vi "公式复合写入.vi"(8 "公式":cluster{"X^2":dbl, "X":dbl, "b":dbl}, 9 "量程下拉列表":enum16{"低量程", "高量程"}(ring), 10 "测量模式":T1(ring), 11 "参数下拉列表":u16(ring) items=["总氮"=2]) -> ()   [LabVIEW 2016, in "斯坦道总磷总氮.lvlib"]
uses:
  <vilib>/Utility/miscctls.llb/LVPointTypeDef.ctl
panel:
  in  "读取":bool
  in  "一键写入":bool=TRUE
  out "连接的字符串":string
  in  "关闭":bool
  in  "写入":bool
  # "请选择要写入的参数"
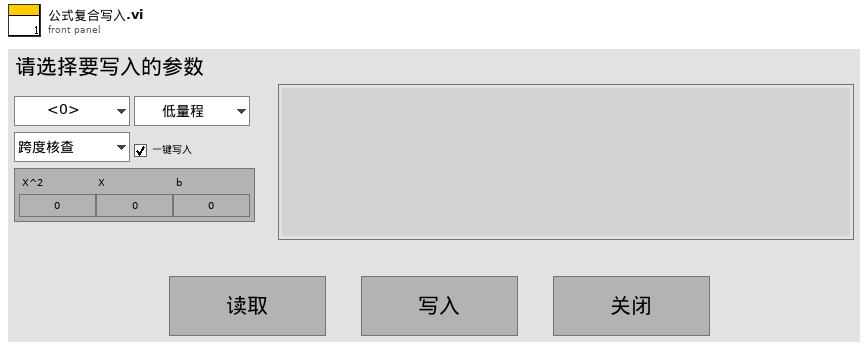
[diagram p1: front panel]
types:
  T1 = enum16{"跨度核查", "水样测量", "零点核查", "标样核查", "加标回收", "快捷测试", "空白校准", "标样校准"}
  T2 = typedef "LVPointTypeDef.ctl" = cluster{"Horizontal":i16, "Vertical":i16}
  T3 = cluster{"系统时间":timestamp, "工作状态":u16, "测量模式":enum16{"待机", "连续模式", "周期模式", "定点模式", "受控模式", "手动模式"}, "告警代码":u16, "故障代码":u16, "日志代码":u16, "软件版本":u16, "F0":sgl, "F1":sgl, "F2":sgl, "F3":sgl, "T":sgl, "H":sgl, "id":u16, "flowid":u16, "量程":u16, "总磷控温温度1":sgl, "营养盐控温温度2":sgl, "ADC":sgl}
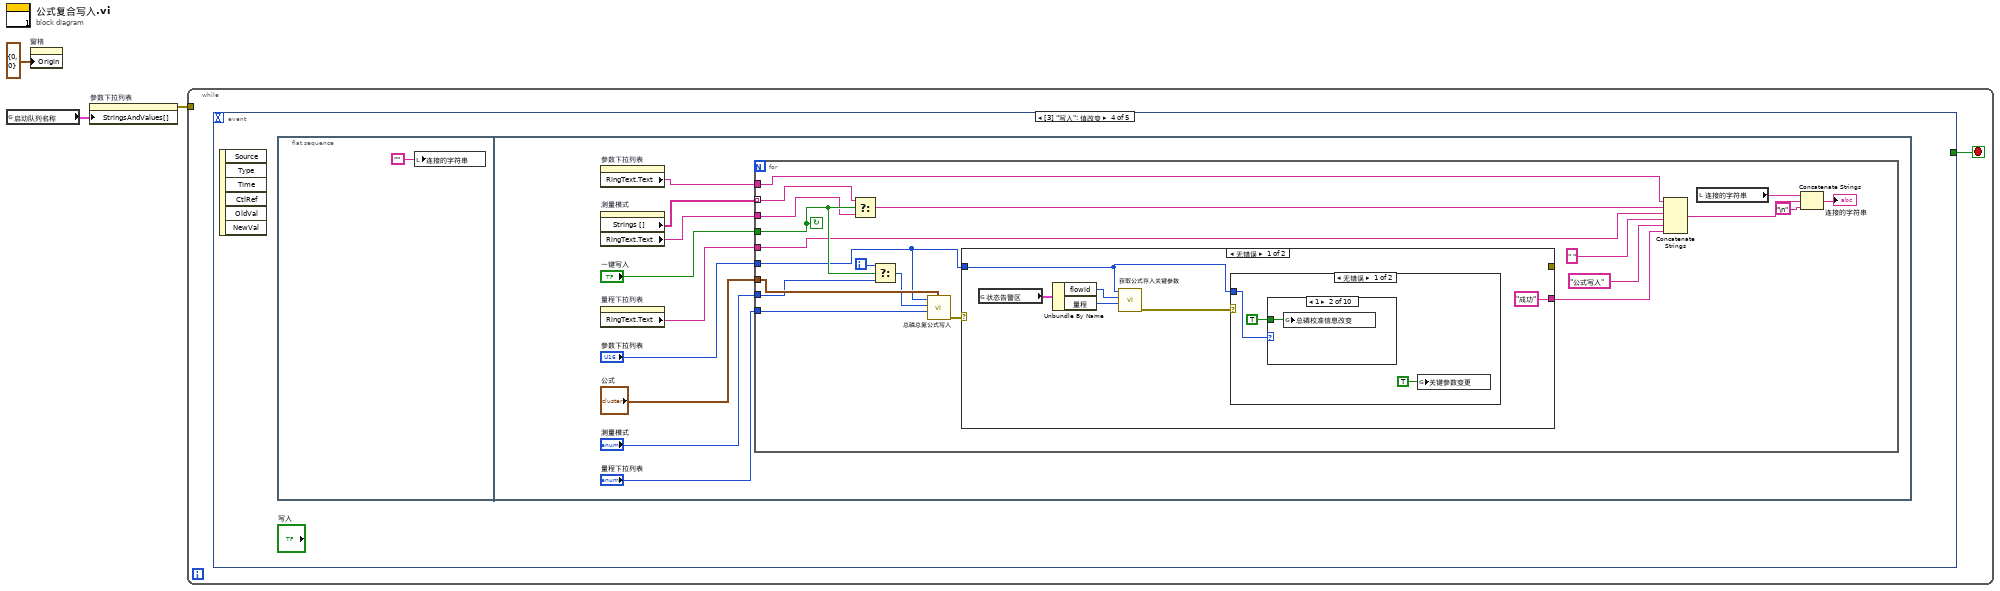
[diagram p0: block diagram]
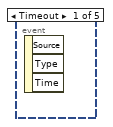
[diagram p2: hidden frame]
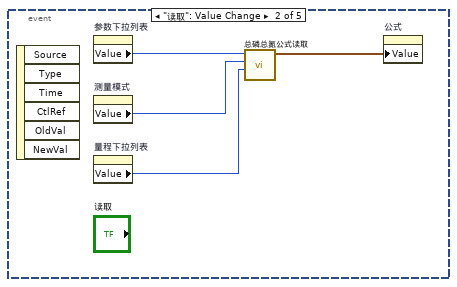
[diagram p3: hidden frame]
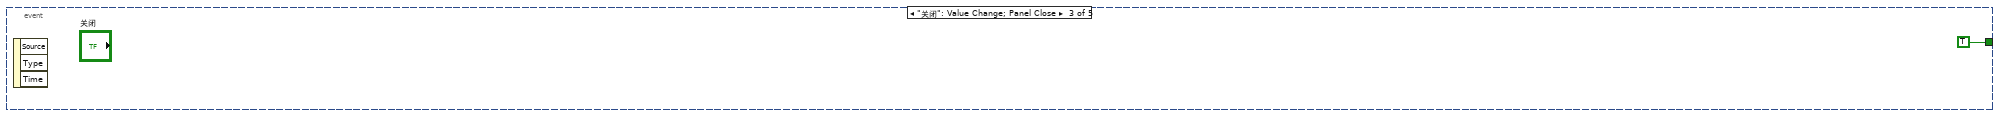
[diagram p4: hidden frame]
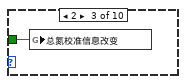
[diagram p6: hidden frame]
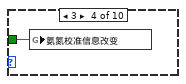
[diagram p7: hidden frame]
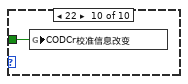
[diagram p13: hidden frame]
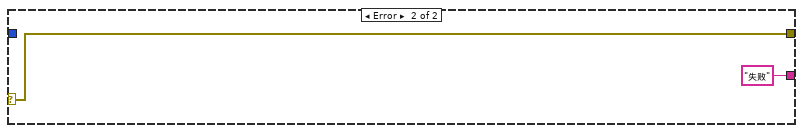
[diagram p15: hidden frame]
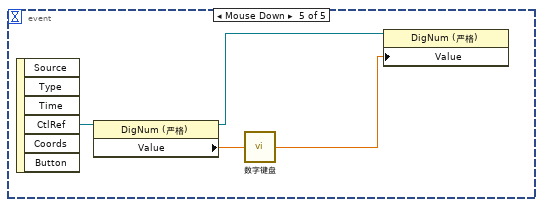
[diagram p16: hidden frame]
diagram:
  n1 = global read "model config var.vi" "启动队列名称"() -> (w2:cluster{"String":string, "Value":u16}[])
  n2 = property on="窗格" class="Pane"("Origin"=T2 {"Horizontal"=0, "Vertical"=0} ("原点")) -> ()  [unwired: 2 in, 2 out]
  n3 = property on="参数下拉列表" class="Ring (严格)"("StringsAndValues[]"=w2) -> (error out=w1:errorcluster)  [unwired: 2 in, 1 out]
  n4 = while {
    tunnel: w1 -> [_]
    stop <- w4 stop-if-true
    n5 = event shown="[3] \"写入\": 值改变" {
      selector: _ -> [_ _ _ _ _]
      dyn-events: _ -> [_ _ _ _ _]
      timeout: _ -> [_ _ _ _ _]
      tunnel: [_ _ TRUE _ _] -> w4
      event Timeout {
        n6 = event-data() -> ()  [unwired: 1 in, 3 out]
      }
      event "读取": Value Change {
        n7 = event-data() -> ()  [unwired: 1 in, 6 out]
        n8 = property on="参数下拉列表" class="Ring (严格)"() -> ("Value"=w8:u16)  [unwired: 2 in, 2 out]
        n9 = property on="测量模式" class="Enum (严格)"() -> ("Value"=w7:T1)  [unwired: 2 in, 2 out]
        n10 = property on="量程下拉列表" class="Enum (严格)"() -> ("Value"=w6:enum16{"低量程", "高量程"})  [unwired: 2 in, 2 out]
        n11 = call "总磷总氮公式读取.vi"("量程"=w6, "测量模式"=w7, "测量参数"=w8) -> ("公式"=w5:cluster{"X^2":dbl, "X":dbl, "b":dbl})  [unwired: 7 in, 1 out]
        n12 = property on="公式" class="Clust (严格)"("Value"=w5) -> ()  [unwired: 2 in, 2 out]
      }
      event "关闭": Value Change; Panel Close {
        n13 = event-data() -> ()  [unwired: 1 in, 3 out]
      }
      event "写入": Value Change {
        n14 = event-data() -> ()  [unwired: 1 in, 6 out]
        n15 = flat-sequence {
          frame #0 {
            n16 = local write "连接的字符串"("") -> ()
          }
          frame #1 {
            n17 = property on="参数下拉列表" class="Ring (严格)"() -> ("RingText.Text"=w12:string)  [unwired: 2 in, 2 out]
            n18 = property on="测量模式" class="Enum (严格)"() -> ("Strings []"=w16:string[], "RingText.Text"=w15:string)  [unwired: 2 in, 2 out]
            n19 = property on="量程下拉列表" class="Enum (严格)"() -> ("RingText.Text"=w11:string)  [unwired: 2 in, 2 out]
            n20 = for {
              tunnel: "公式" -> [w39]
              tunnel: "参数下拉列表" -> [w20]
              tunnel: "量程下拉列表" -> [w38]
              tunnel: w16 -> [w32] mode=indexing
              tunnel: w15 -> [w31]
              tunnel: "一键写入" -> [w33]
              tunnel: "测量模式" -> [w35]
              tunnel: w12 -> [w23]
              tunnel: w11 -> [w21]
              i -> [w36]
              stop <- w33 continue-if-true
              n21 = Select(t=w32, s=w33, f=w31) -> (s? t:f=w25:string)
              n22 = Select(t=w36, s=w33, f=w35) -> (s? t:f=w34:i32)
              n23 = call "总磷总氮公式写入.vi"("公式"=w39, "量程"=w38, "测量模式"=w34, "测量参数"=w20) -> ("error out"=w37:errorcluster)  [unwired: 7 in]
              n24 = case shown="无错误" w37 {
                selector: w37 -> [_ w54]
                tunnel: [_ w54] -> _
                tunnel: ["成功" "失败"] -> w24
                tunnel: w20 -> [w41 _]
                frame No Error {
                  n25 = global read "VAR总磷总氮全局变量.vi" "状态告警区"() -> (w42:T3)
                  n26 = Unbundle By Name(w42) -> ("flowid"=w44:u16, "量程"=w43:u16)
                  n27 = call "获取公式存入关键参数.vi"("量程"=w43, "flowid"=w44, "id"=w41) -> ("error out"=w40:errorcluster)  [unwired: 7 in, 1 out]
                  n28 = case shown="无错误" w40 {
                    tunnel: w41 -> [w46 _]
                    frame No Error {
                      n29 = case shown="1" w46 {
                        tunnel: TRUE ("总磷关键参数改变") -> [_ w49 w50 w51 _ _ _ _ _ w52]
                        frame 0, Default {
                        }
                        frame 1 {
                          n30 = global write "VAR总磷总氮全局变量.vi" "总磷校准信息改变"(w49) -> ()
                        }
                        frame 2 {
                          n31 = global write "VAR总磷总氮全局变量.vi" "总氮校准信息改变"(w50) -> ()
                        }
                        frame 3 {
                          n32 = global write "VAR总磷总氮全局变量.vi" "氨氮校准信息改变"(w51) -> ()
                        }
                        frame 4 {
                        }
                        frame 5 {
                        }
                        frame 6 {
                        }
                        frame 7 {
                        }
                        frame 8 {
                        }
                        frame 22 {
                          n33 = global write "VAR总磷总氮全局变量.vi" "CODCr校准信息改变"(w52) -> ()
                        }
                      }
                      n34 = global write "VAR总磷总氮全局变量.vi" "关键参数变更"(TRUE ("关键参数变更")) -> ()
                    }
                    frame Error {
                    }
                  }
                }
                frame Error {
                }
              }
              n35 = Concatenate Strings(w23, w25, w21, " " ("字符串"), "公式写入", w24) -> (w29:string)
              n36 = local read "连接的字符串"() -> (w26:string)
              n37 = Concatenate Strings(w26, w29, "\n") -> (→"连接的字符串":string)
            }
          }
        }
      }
      event "公式.X^2", "公式.X", "公式.b": Mouse Down {
        n38 = event-data() -> ("CtlRef"=w58:refnum<vi>)  [unwired: 1 in, 5 out]
        n39 = property class="DigNum (严格)"(reference=w58) -> (reference out=w55:refnum<vi>, "Value"=w57:dbl)  [unwired: 1 in, 1 out]
        n40 = call "数字键盘.vi"("OldNumber"=w57) -> ("NewNumber"=w56:dbl)
        n41 = property class="DigNum (严格)"(reference=w55, "Value"=w56) -> ()  [unwired: 1 in, 2 out]
      }
    }
  }
